vi "Read Disabled Items.vi"(9 "NamedNumeric in":refnum<class "NamedNumeric.lvclass">) -> (3 "NamedNumeric out":refnum<class "NamedNumeric.lvclass">, 4 "Disabled Items":i32[](array[numeric]))   [LabVIEW 2014, in "Raspberry Pi Compatible Compiler for LabVIEW.lvlib" / "NamedNumeric.lvclass"]
uses:
  NamedNumeric.lvclass
  NamedNumeric.lvclass/NamedNumeric.ctl
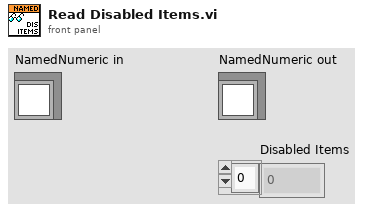
[diagram p1: front panel]
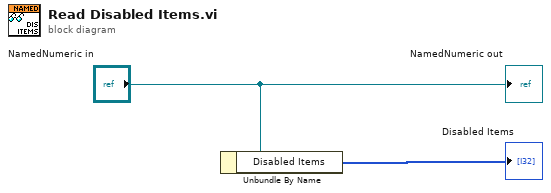
[diagram p0: block diagram]
diagram:
  n1 = Unbundle By Name("NamedNumeric in") -> ("Disabled Items"=→"Disabled Items":i32[])
  "NamedNumeric out" <- "NamedNumeric in"
